vi "Update Test Status.vi"(8 "error in (no error)":errorcluster, 11 "Logger in.lvclass":refnum<class "Logger.lvclass">) -> (0 "error out":errorcluster, 3 "Logger out.lvclass":refnum<class "Logger.lvclass">)   [LabVIEW 2024, in "Logger.lvclass"]
uses:
  Logger.lvclass
  Logger.lvclass/Logger.ctl
  <vilib>/Skyline/Tag/Shared/typedefs/TagProperty.ctl
  <vilib>/Skyline/Tag/Wrapper/Wrapper_class/Generate Tag Cluster (String) 2.vi
  <vilib>/Skyline/Tag/Wrapper/Wrapper_class/Generate Tag Cluster Core 2.vi
  <vilib>/Skyline/Tag/Wrapper/Wrapper_class/NI Skyline Tag.lvclass
  <vilib>/Skyline/Tag/Shared/NI Skyline Tag.lvlib
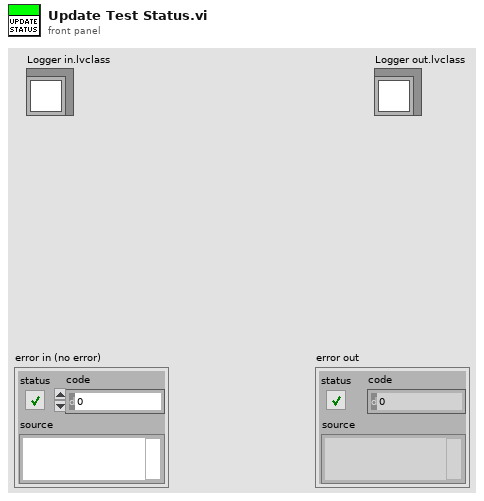
[diagram p1: front panel]
types:
  T1 = typedef "NI Skyline Tag.lvlib/TagProperty.ctl" = cluster{"key":string, "value":string}
  T2 = cluster{"Tag Units":string, "Tag Path":string, "Tag Reference":refnum<class "NI Skyline Tag.lvclass">}[]
  T3 = typedef "NI Skyline Tag.lvclass/Tag Value Cluster Wrapper.ctl" = cluster{"Configuration":refnum<class "NI Skyline Configuration.lvclass">, "Tag Cluster":T4}
  T4 = typedef "NI Skyline Tag.lvlib/Tag Value Cluster.ctl" = cluster{"Path":string, "Workspace ID":string, "Data Type":T5, "Value":string, "Time Stamp":timestamp}
  T5 = typedef "NI Skyline Tag.lvlib/DataType.ctl" = enum32{"Double", "I32", "String", "Boolean", "U64", "Timestamp"}
  T6 = cluster{"Tag Units":string, "Tag Path":string, "Tag Reference":refnum<class "NI Skyline Tag.lvclass">}
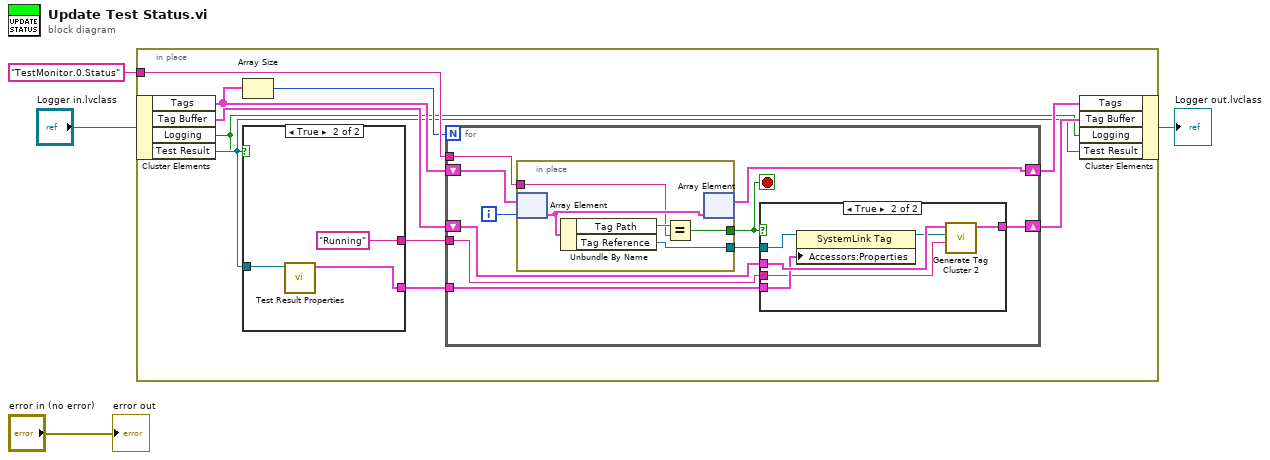
[diagram p0: block diagram]
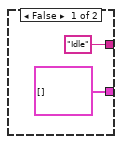
[diagram p2: hidden frame]
diagram:
  n1 = in-place {
    in-place-border: "TestMonitor.0.Status" ("Tag Path") -> [w14]
    n2 = in-place-cluster #1("Logger in.lvclass") -> ("Tags"=w11:T2, "Tag Buffer"=w10:T3[], "Logging"=w5:bool, "Test Result"=w6:refnum<class "NI SystemLink Test Result.lvclass">)
    n3 = Array Size(array=w11) -> (size(s)=w12:i32)
    n4 = case shown="True" w5 {
      tunnel: w6 -> [_ w19]
      tunnel: [T1[] [] ("Array") w18] -> w8
      tunnel: ["Idle" "Running"] -> w7
      frame False {
      }
      frame True {
        n5 = call "Test Result Properties.vi"("NI SystemLink Test Result in"=w19) -> ("Array"=w18:T1[])  [unwired: 10 in]
      }
    }
    n6 = for {
      N: w12 -> [_]
      tunnel: w14 -> [w29]
      shift-right: [w24] -> w13
      shift-left: w11 -> [w28]
      shift-right: [w22] -> w9
      shift-left: w10 -> [w23]
      tunnel: w8 -> [w21]
      tunnel: w7 -> [w20]
      i -> [w27]
      stop <- w26 stop-if-true
      n7 = in-place {
        in-place-border: w29 -> [w37]
        in-place-border: [w39] -> w26
        in-place-border: [w41] -> w25
        n8 = in-place-array #2(w28, w27) -> (w40:T6)
        n9 = Unbundle By Name(w40) -> ("Tag Path"=w38:string, "Tag Reference"=w41:refnum<class "NI Skyline Tag.lvclass">)
        n10 = Equal?(x=w38, y=w37) -> (x = y?=w39:bool)
        n11 = in-place-array #2(w40) -> (w24:T2)  [unwired: 1 out]
      }
      n12 = case shown="True" w26 {
        tunnel: w25 -> [_ w34]
        tunnel: w23 -> [w30 w36]
        tunnel: [w30 w35] -> w22
        tunnel: w21 -> [_ w32]
        tunnel: w20 -> [_ w31]
        frame False {
        }
        frame True {
          n13 = property on="Property Node" class="SystemLink Tag"(reference=w34, "Accessors:Properties"=w32) -> (reference out=w33:refnum<class "NI Skyline Tag.lvclass">)  [unwired: 1 in, 1 out]
          n14 = call-poly <vilib>:"Generate Tag Cluster 2.vi"("value"=w31, "tag in"=w33, "tag clusters in"=w36) -> ("tag clusters out"=w35:T3[])  [unwired: 6 in, 2 out]
        }
      }
    }
    n15 = in-place-cluster #1("Tags"=w13, "Tag Buffer"=w9, "Logging"=w5, "Test Result"=w6) -> (→"Logger out.lvclass":refnum<class "Logger.lvclass">)
  }
  "error out" <- "error in (no error)"
